vi "Save Load Cycle Setting.vi"(8 "error in (no error)":errorcluster, 10 "Operation (0: Save)":u16(ring) items=["Save", "Load"], 11 "Actor_AFG in":refnum<class "Actor_AFG.lvclass">) -> (0 "error out":errorcluster, 3 "Actor_AFG out":refnum<class "Actor_AFG.lvclass">)   [LabVIEW 2020, in "Actor_AFG.lvlib" / "Actor_AFG.lvclass"]
uses:
  Actor_AFG.lvclass
  Actor_AFG.lvclass/Actor_AFG.ctl
  <instrlib>/Tektronix AFG 3000 Series/Tektronix AFG 3000 Series.lvlib
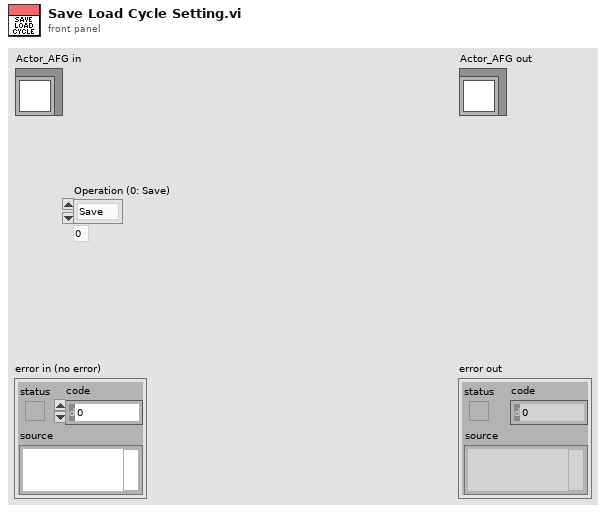
[diagram p1: front panel]
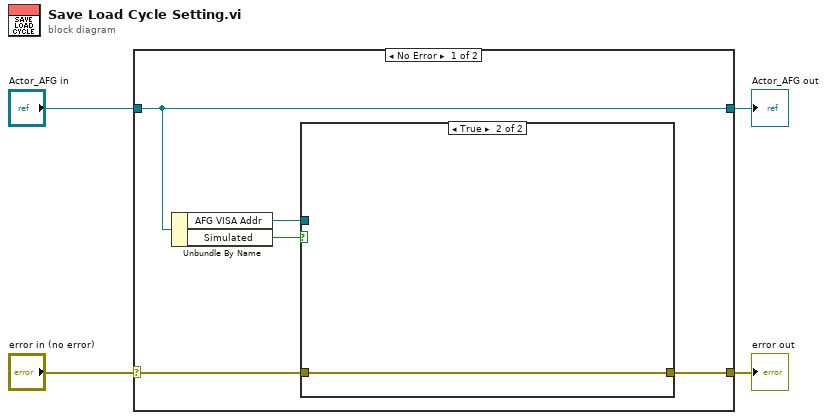
[diagram p0: block diagram]
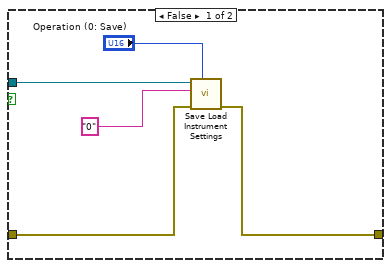
[diagram p2: hidden frame]
diagram:
  n1 = case shown="No Error" "error in (no error)" {
    selector: "error in (no error)" -> [w6 w17]
    tunnel: [w5 w17] -> w3
    tunnel: [w9 w16] -> w1
    tunnel: "Actor_AFG in" -> [w9 w16]
    frame No Error {
      n2 = Unbundle By Name(w9) -> ("AFG VISA Addr"=w7:refnum<visa-resource-name>, "Simulated"=w8:bool)
      n3 = case shown="True" w8 {
        tunnel: w7 -> [w14 _]
        tunnel: w6 -> [w12 w15]
        tunnel: [w11 w15] -> w5
        frame False {
          n4 = call <instrlib>:"Save Load Instrument Settings.vi"("Operation (0: Save)"="Operation (0: Save)", "error in (no error)"=w12, "Setting File Name (Setting0.TFS)"="0", "VISA resource name"=w14) -> ("error out"=w11:errorcluster)  [unwired: 6 in, 1 out]
        }
        frame True {
        }
      }
    }
    frame Error {
    }
  }
  "error out" <- w3
  "Actor_AFG out" <- w1
